vi "SMD7615 UDP Reset Position.vi"(8 "error in (no error)":errorcluster, 10 "IP":string="192.168.1.30", 11 "connection ID in":refnum<k16>) -> (0 "error out":errorcluster, 3 "connection ID out":refnum<k16>)   [LabVIEW 2016, in "SMD-7615.lvlib" / "eSCL.lvlib"]
uses:
  eSCL.lvlib
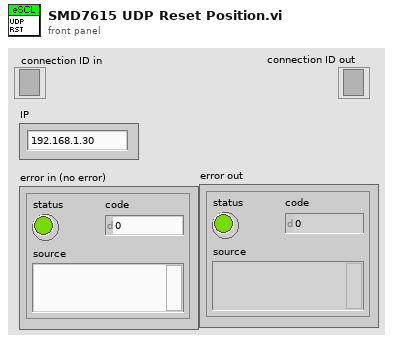
[diagram p1: front panel]
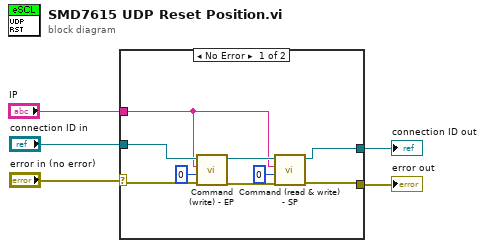
[diagram p0: block diagram]
diagram:
  n1 = case shown="No Error" "error in (no error)" {
    selector: "error in (no error)" -> [w11 w15]
    tunnel: "connection ID in" -> [w12 w16]
    tunnel: [w13 w16] -> w3
    tunnel: [w14 w15] -> w2
    tunnel: "IP" -> [w6 _]
    frame No Error {
      n2 = call "Command (write) - EP.vi"("error in (no error)"=w11, "Encoder Position"=0, "IP"=w6, "connection ID in"=w12) -> ("error out"=w8:errorcluster, "connection ID out"=w7:refnum<k16>)  [unwired: 6 in]
      n3 = call "Command (read & write) - SP.vi"("error in (no error)"=w8, "Position"=0, "IP"=w6, "connection ID in"=w7) -> ("error out"=w14:errorcluster, "connection ID out"=w13:refnum<k16>)  [unwired: 5 in, 1 out]
    }
    frame Error {
    }
  }
  "connection ID out" <- w3
  "error out" <- w2
